vi "Solve2.vi"(8 "Error In":errorcluster, 11 "object in":refnum<class "2021_2.lvclass">) -> (0 "Error Out":errorcluster, 2 "Result":u64, 3 "object out":refnum<class "2021_2.lvclass">)   [LabVIEW 2020, in "2021_2.lvclass"]
uses:
  2021_2.lvclass
  2021_2.lvclass/2021_2.ctl
panel:
  out "Depth":i32
  out "Aim":i32
  out "Forward":i32
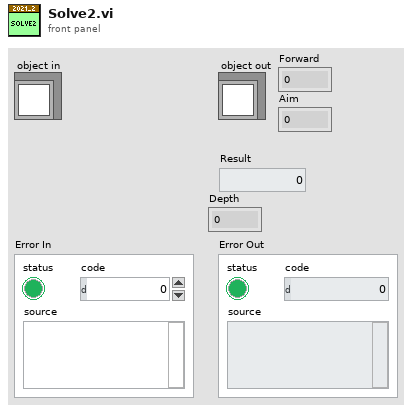
[diagram p1: front panel]
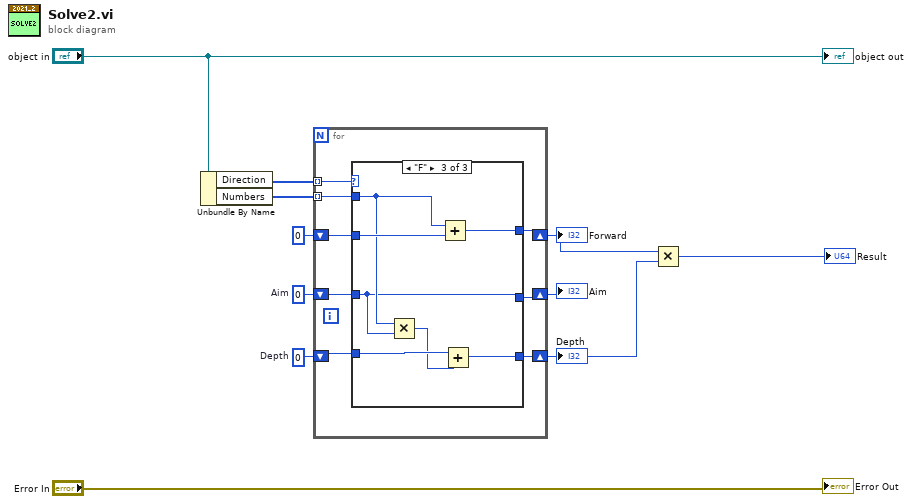
[diagram p0: block diagram]
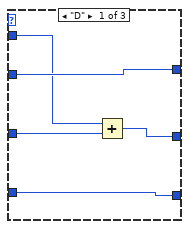
[diagram p2: hidden frame]
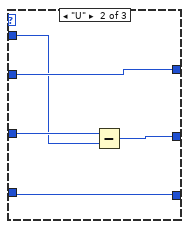
[diagram p3: hidden frame]
diagram:
  w2 = 0  # Depth
  w7 = 0  # Aim
  n1 = Unbundle By Name("object in") -> ("Direction"=w6:enum16{"F", "D", "U"}[], "Numbers"=w8:i32[])
  n2 = for {
    tunnel: w8 -> [w14] mode=indexing
    shift-right: [w18] -> w3
    shift-left: w7 -> [w19]
    tunnel: w6 -> [w17] mode=indexing
    shift-right: [w16] -> w4
    shift-left: 0 -> [w15]
    shift-right: [w12] -> w1
    shift-left: w2 -> [w13]
    n3 = case shown="\"F\"" w17 {
      tunnel: w19 -> [w21 w29 w31]
      tunnel: [w24 w26 w31] -> w18
      tunnel: w15 -> [w23 w28 w35]
      tunnel: [w23 w28 w36] -> w16
      tunnel: w14 -> [w22 w27 w32]
      tunnel: w13 -> [w20 w25 w33]
      tunnel: [w20 w25 w34] -> w12
      frame "D" {
        n4 = Add(x=w22, y=w21) -> (x+y=w24:i32)
      }
      frame "U" {
        n5 = Subtract(x=w29, y=w27) -> (x-y=w26:i32)
      }
      frame "F" {
        n6 = Multiply(x=w32, y=w31) -> (x*y=w30:i32)
        n7 = Add(x=w32, y=w35) -> (x+y=w36:i32)
        n8 = Add(x=w33, y=w30) -> (x+y=w34:i32)
      }
    }
  }
  "Forward" <- w4
  "Aim" <- w3
  "Depth" <- w1
  n9 = Multiply(x=w4, y=w1) -> (x*y=→"Result":i32)
  "Error Out" <- "Error In"
  "object out" <- "object in"
